vi "Convert file.vi"(8 "error in (no error)":errorcluster, 9 "file out":path, 10 "file in":path, 11 "DAQMH121119OrcaFlash in":refnum<class "DAQOrcaFlash.lvclass">) -> (0 "error out":errorcluster, 3 "DAQMH121119OrcaFlash out":refnum<class "DAQOrcaFlash.lvclass">)   [LabVIEW 2012, in "DAQOrcaFlash.lvclass"]
uses:
  DAQOrcaFlash.lvclass
  DAQOrcaFlash.lvclass/DAQOrcaFlash.ctl
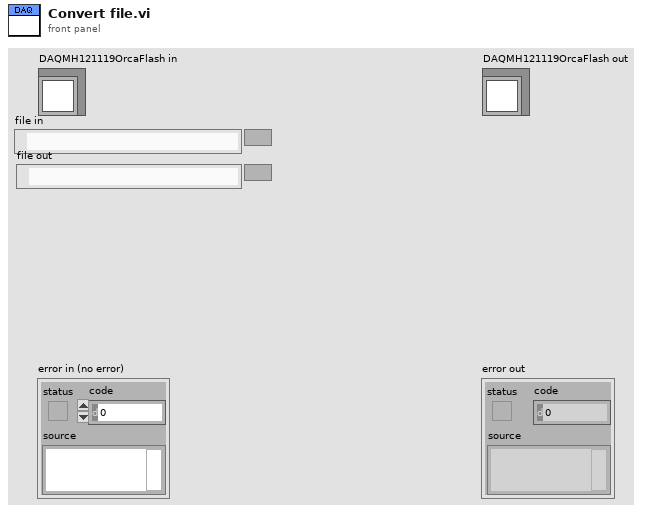
[diagram p1: front panel]
types:
  T1 = typedef "Image Type" = u32
  T2 = typedef "IMAQ Image.ctl" = refnum<image>
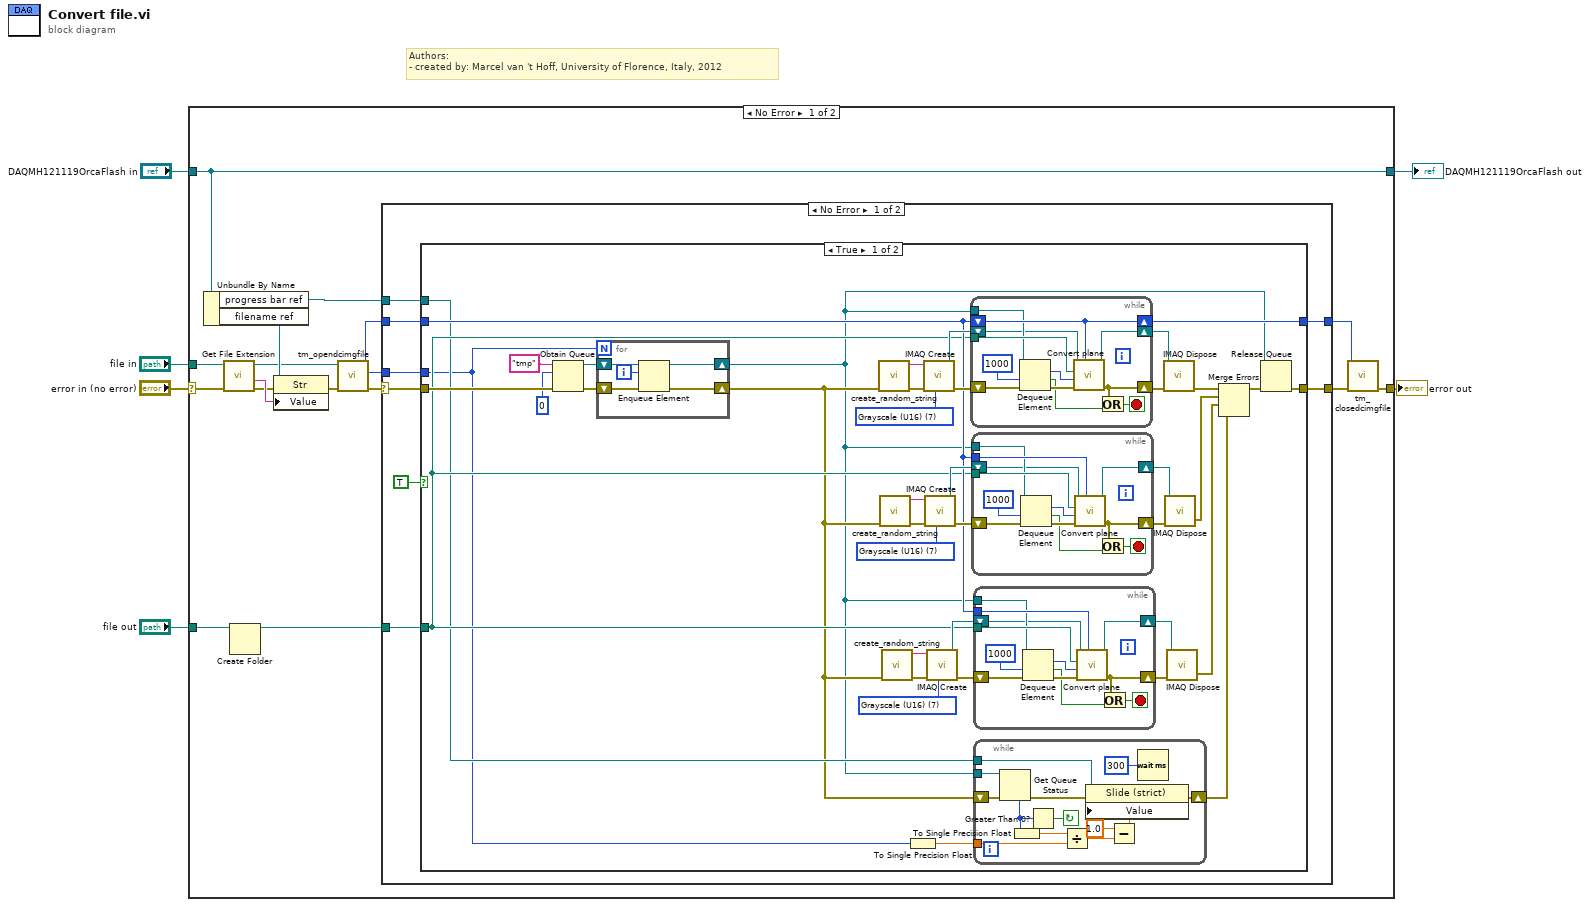
[diagram p0: block diagram]
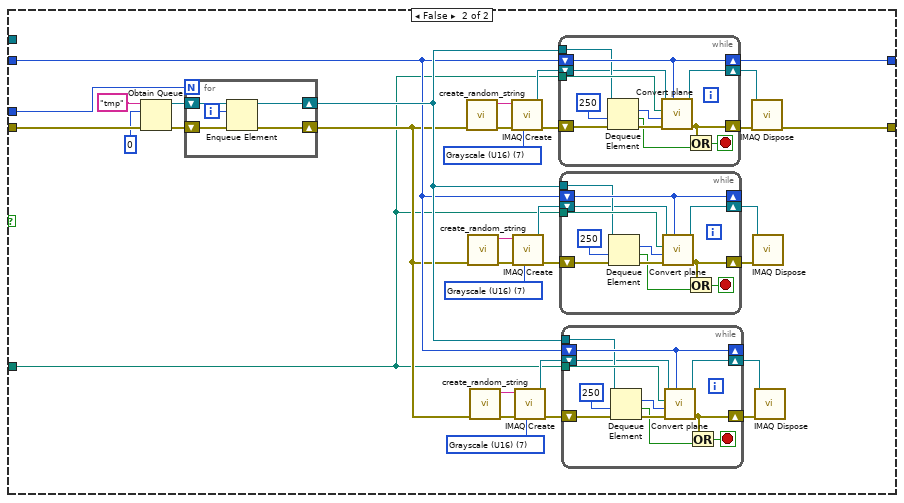
[diagram p2: hidden frame]
diagram:
  # "Authors: \n- created by: Marcel van 't Hoff, University of Florence, Italy, 2012"
  n1 = case shown="No Error" "error in (no error)" {
    selector: "error in (no error)" -> [w12 w203]
    tunnel: [w13 w203] -> w5
    tunnel: [w23 w202] -> w1
    tunnel: "DAQMH121119OrcaFlash in" -> [w23 w202]
    tunnel: "file in" -> [w11 _]
    tunnel: "file out" -> [w10 _]
    frame No Error {
      n2 = Unbundle By Name(w23) -> ("progress bar ref"=w19:refnum<vi>, "filename ref"=w22:refnum<vi>)
      n3 = call <vilib>:"Get File Extension.vi"("error in (no error)"=w12, "file"=w11) -> ("error out"=w20:errorcluster, "filename without extension"=w21:string, "dup file"=w7:path)  [unwired: 6 in, 1 out]
      n4 = Create Folder(path (use dialog)=w10) -> (created path=w9:path)  [unwired: 2 in, 2 out]
      n5 = property class="Str"(reference=w22, error in=w20, "Value"=w21) -> (error out=w8:errorcluster)  [unwired: 1 out]
      n6 = call <userlib>:"tm_opendcimgfile.vi"("error in (no error)"=w8, "Path"=w7) -> ("error out"=w16:errorcluster, "Total Frames"=w18:i32, "File Handle"=w17:u32)  [unwired: 7 in]
      n7 = case shown="No Error" w16 {
        selector: w16 -> [w31 w201]
        tunnel: w17 -> [w27 w200]
        tunnel: [w29 w201] -> w14
        tunnel: w18 -> [w28 _]
        tunnel: w9 -> [w26 _]
        tunnel: w19 -> [w24 _]
        tunnel: [w30 w200] -> w15
        frame No Error {
          n8 = case shown="True" TRUE {
            tunnel: w31 -> [w65 w152]
            tunnel: [w64 w151] -> w30
            tunnel: [w33 w150] -> w29
            tunnel: w28 -> [w40 w143]
            tunnel: w27 -> [w48 w132]
            tunnel: w26 -> [w47 w130]
            tunnel: w24 -> [w42 _]
            frame True {
              w50 = T1 7 items=["Grayscale (U8)", "Grayscale (I16)", "Grayscale (SGL)", "Complex (CSG)", "RGB (U32)", "HSL (U32)", "RGB (U64)", "Grayscale (U16)"] ("Image Type")
              w62 = T1 7 items=["Grayscale (U8)", "Grayscale (I16)", "Grayscale (SGL)", "Complex (CSG)", "RGB (U32)", "HSL (U32)", "RGB (U64)", "Grayscale (U16)"] ("Image Type")
              w67 = T1 7 items=["Grayscale (U8)", "Grayscale (I16)", "Grayscale (SGL)", "Complex (CSG)", "RGB (U32)", "HSL (U32)", "RGB (U64)", "Grayscale (U16)"] ("Image Type")
              n9 = Obtain Queue(name (unnamed)="tmp", element data type=0, error in (no error)=w65) -> (queue out=w43:refnum<queue>, error out=w46:errorcluster)  [unwired: 2 in, 1 out]
              n10 = for {
                N: w40 -> [_]
                shift-right: [w86] -> w41
                shift-left: w46 -> [w89]
                shift-right: [w85] -> w32
                shift-left: w43 -> [w88]
                i -> [w87]
                n11 = Enqueue Element(queue=w88, element=w87, error in (no error)=w89) -> (queue out=w85:refnum<queue>, error out=w86:errorcluster)  [unwired: 1 in, 1 out]
              }
              n12 = call "create_random_string.vi"("error in (no error)"=w41) -> ("error out"=w69:errorcluster, "random string"=w68:string)  [unwired: 9 in]
              n13 = call "create_random_string.vi"("error in (no error)"=w41) -> ("error out"=w60:errorcluster, "random string"=w61:string)  [unwired: 9 in]
              n14 = call "create_random_string.vi"("error in (no error)"=w41) -> ("error out"=w52:errorcluster, "random string"=w51:string)  [unwired: 9 in]
              n15 = To Single Precision Float(number=w40) -> (single precision float=w39:sgl)
              n16 = call "IMAQ Create"("Image Name"=w68, "Image Type"=w67, "error in (no error)"=w69) -> ("New Image"=w70:T2, "error out"=w66:errorcluster)  [unwired: 2 in]
              n17 = call "IMAQ Create"("Image Name"=w61, "Image Type"=w62, "error in (no error)"=w60) -> ("New Image"=w59:T2, "error out"=w63:errorcluster)  [unwired: 2 in]
              n18 = call "IMAQ Create"("Image Name"=w51, "Image Type"=w50, "error in (no error)"=w52) -> ("New Image"=w53:T2, "error out"=w49:errorcluster)  [unwired: 2 in]
              n19 = while {
                tunnel: w47 -> [w125]
                shift-right: [w116] -> w57
                shift-left: w66 -> [w121]
                shift-right: [w124] -> w71
                shift-left: w70 -> [w119]
                shift-right: [w123] -> w64
                shift-left: w48 -> [w123]
                tunnel: w32 -> [w122]
                stop <- w114 stop-if-true
                n20 = Dequeue Element(queue=w122, timeout in ms (-1)=1000, error in (no error)=w121) -> (element=w120:i32, timed out?=w115:bool, error out=w117:errorcluster)  [unwired: 1 out]
                n21 = call "Convert plane.vi"("File Handle"=w123, "error in (no error)"=w117, "Frame Index"=w120, "file in"=w125, "Image in"=w119) -> ("error out"=w116:errorcluster, "Image out"=w124:T2)  [unwired: 5 in]
                n22 = Or(x=w116, y=w115) -> (x .or. y?=w114:bool)
              }
              n23 = while {
                tunnel: w47 -> [w113]
                shift-right: [w102] -> w56
                shift-left: w63 -> [w109]
                shift-right: [w112] -> w58
                shift-left: w59 -> [w106]
                tunnel: w32 -> [w110]
                tunnel: w48 -> [w111]
                stop <- w103 stop-if-true
                n24 = Dequeue Element(queue=w110, timeout in ms (-1)=1000, error in (no error)=w109) -> (element=w107:i32, timed out?=w104:bool, error out=w108:errorcluster)  [unwired: 1 out]
                n25 = call "Convert plane.vi"("File Handle"=w111, "error in (no error)"=w108, "Frame Index"=w107, "file in"=w113, "Image in"=w106) -> ("error out"=w102:errorcluster, "Image out"=w112:T2)  [unwired: 5 in]
                n26 = Or(x=w102, y=w104) -> (x .or. y?=w103:bool)
              }
              n27 = while {
                tunnel: w47 -> [w101]
                shift-right: [w90] -> w55
                shift-left: w49 -> [w97]
                shift-right: [w100] -> w54
                shift-left: w53 -> [w94]
                tunnel: w32 -> [w98]
                tunnel: w48 -> [w99]
                stop <- w91 stop-if-true
                n28 = Dequeue Element(queue=w98, timeout in ms (-1)=1000, error in (no error)=w97) -> (element=w95:i32, timed out?=w92:bool, error out=w96:errorcluster)  [unwired: 1 out]
                n29 = call "Convert plane.vi"("File Handle"=w99, "error in (no error)"=w96, "Frame Index"=w95, "file in"=w101, "Image in"=w94) -> ("error out"=w90:errorcluster, "Image out"=w100:T2)  [unwired: 5 in]
                n30 = Or(x=w90, y=w92) -> (x .or. y?=w91:bool)
              }
              n31 = while {
                tunnel: w32 -> [w84]
                tunnel: w42 -> [w82]
                shift-right: [w79] -> w36
                shift-left: w41 -> [w80]
                tunnel: w39 -> [w77]
                stop <- w83 continue-if-true
                n32 = Get Queue Status(queue=w84, error in (no error)=w80) -> (error out=w81:errorcluster, # elements in queue=w78:i32)  [unwired: 1 in, 6 out]
                n33 = To Single Precision Float(number=w78) -> (single precision float=w76:sgl)
                n34 = Greater Than 0?(x=w78) -> (x > 0?=w83:bool)
                n35 = Divide(x=w76, y=w77) -> (x/y=w74:sgl)
                n36 = Subtract(x=sgl 1.0, y=w74) -> (x-y=w72:sgl)
                n37 = property class="Slide (strict)"(reference=w82, error in=w81, "Value"=w72) -> (error out=w79:errorcluster)  [unwired: 1 out]
                n38 = Wait (ms)(milliseconds to wait=u32 300) -> ()  [unwired: 1 out]
              }
              n39 = call "IMAQ Dispose"("Image"=w71, "error in (no error)"=w57) -> ("error out"=w35:errorcluster)  [unwired: 4 in]
              n40 = call "IMAQ Dispose"("Image"=w58, "error in (no error)"=w56) -> ("error out"=w38:errorcluster)  [unwired: 4 in]
              n41 = call "IMAQ Dispose"("Image"=w54, "error in (no error)"=w55) -> ("error out"=w37:errorcluster)  [unwired: 4 in]
              n42 = Merge Errors(w35, w38, w37, w36) -> (w34:errorcluster)
              n43 = Release Queue(queue=w32, error in (no error)=w34) -> (error out=w33:errorcluster)  [unwired: 1 in, 2 out]
            }
            frame False {
              w135 = T1 7 items=["Grayscale (U8)", "Grayscale (I16)", "Grayscale (SGL)", "Complex (CSG)", "RGB (U32)", "HSL (U32)", "RGB (U64)", "Grayscale (U16)"] ("Image Type")
              w148 = T1 7 items=["Grayscale (U8)", "Grayscale (I16)", "Grayscale (SGL)", "Complex (CSG)", "RGB (U32)", "HSL (U32)", "RGB (U64)", "Grayscale (U16)"] ("Image Type")
              w154 = T1 7 items=["Grayscale (U8)", "Grayscale (I16)", "Grayscale (SGL)", "Complex (CSG)", "RGB (U32)", "HSL (U32)", "RGB (U64)", "Grayscale (U16)"] ("Image Type")
              n44 = Obtain Queue(name (unnamed)="tmp", element data type=0, error in (no error)=w152) -> (queue out=w126:refnum<queue>, error out=w129:errorcluster)  [unwired: 2 in, 1 out]
              n45 = for {
                N: w143 -> [_]
                shift-right: [w160] -> w131
                shift-left: w129 -> [w163]
                shift-right: [w159] -> w133
                shift-left: w126 -> [w162]
                i -> [w161]
                n46 = Enqueue Element(queue=w162, element=w161, error in (no error)=w163) -> (queue out=w159:refnum<queue>, error out=w160:errorcluster)  [unwired: 1 in, 1 out]
              }
              n47 = call "create_random_string.vi"("error in (no error)"=w131) -> ("error out"=w156:errorcluster, "random string"=w155:string)  [unwired: 9 in]
              n48 = call "create_random_string.vi"("error in (no error)"=w131) -> ("error out"=w146:errorcluster, "random string"=w147:string)  [unwired: 9 in]
              n49 = call "create_random_string.vi"("error in (no error)"=w131) -> ("error out"=w137:errorcluster, "random string"=w136:string)  [unwired: 9 in]
              n50 = call "IMAQ Create"("Image Name"=w155, "Image Type"=w154, "error in (no error)"=w156) -> ("New Image"=w157:T2, "error out"=w153:errorcluster)  [unwired: 2 in]
              n51 = call "IMAQ Create"("Image Name"=w147, "Image Type"=w148, "error in (no error)"=w146) -> ("New Image"=w145:T2, "error out"=w149:errorcluster)  [unwired: 2 in]
              n52 = call "IMAQ Create"("Image Name"=w136, "Image Type"=w135, "error in (no error)"=w137) -> ("New Image"=w138:T2, "error out"=w134:errorcluster)  [unwired: 2 in]
              n53 = while {
                tunnel: w130 -> [w199]
                shift-right: [w190] -> w142
                shift-left: w153 -> [w195]
                shift-right: [w198] -> w158
                shift-left: w157 -> [w193]
                shift-right: [w197] -> w151
                shift-left: w132 -> [w197]
                tunnel: w133 -> [w196]
                stop <- w188 stop-if-true
                n54 = Dequeue Element(queue=w196, timeout in ms (-1)=250, error in (no error)=w195) -> (element=w194:i32, timed out?=w189:bool, error out=w191:errorcluster)  [unwired: 1 out]
                n55 = call "Convert plane.vi"("File Handle"=w197, "error in (no error)"=w191, "Frame Index"=w194, "file in"=w199, "Image in"=w193) -> ("error out"=w190:errorcluster, "Image out"=w198:T2)  [unwired: 5 in]
                n56 = Or(x=w190, y=w189) -> (x .or. y?=w188:bool)
              }
              n57 = while {
                tunnel: w130 -> [w187]
                shift-right: [w176] -> w141
                shift-left: w149 -> [w183]
                shift-right: [w186] -> w144
                shift-left: w145 -> [w180]
                shift-right: [w185] -> _
                shift-left: w132 -> [w185]
                tunnel: w133 -> [w184]
                stop <- w177 stop-if-true
                n58 = Dequeue Element(queue=w184, timeout in ms (-1)=250, error in (no error)=w183) -> (element=w181:i32, timed out?=w178:bool, error out=w182:errorcluster)  [unwired: 1 out]
                n59 = call "Convert plane.vi"("File Handle"=w185, "error in (no error)"=w182, "Frame Index"=w181, "file in"=w187, "Image in"=w180) -> ("error out"=w176:errorcluster, "Image out"=w186:T2)  [unwired: 5 in]
                n60 = Or(x=w176, y=w178) -> (x .or. y?=w177:bool)
              }
              n61 = while {
                tunnel: w130 -> [w175]
                shift-right: [w164] -> w140
                shift-left: w134 -> [w171]
                shift-right: [w174] -> w139
                shift-left: w138 -> [w168]
                shift-right: [w173] -> _
                shift-left: w132 -> [w173]
                tunnel: w133 -> [w172]
                stop <- w165 stop-if-true
                n62 = Dequeue Element(queue=w172, timeout in ms (-1)=250, error in (no error)=w171) -> (element=w169:i32, timed out?=w166:bool, error out=w170:errorcluster)  [unwired: 1 out]
                n63 = call "Convert plane.vi"("File Handle"=w173, "error in (no error)"=w170, "Frame Index"=w169, "file in"=w175, "Image in"=w168) -> ("error out"=w164:errorcluster, "Image out"=w174:T2)  [unwired: 5 in]
                n64 = Or(x=w164, y=w166) -> (x .or. y?=w165:bool)
              }
              n65 = call "IMAQ Dispose"("Image"=w158, "error in (no error)"=w142) -> ("error out"=w150:errorcluster)  [unwired: 4 in]
              n66 = call "IMAQ Dispose"("Image"=w144, "error in (no error)"=w141) -> ()  [unwired: 4 in, 1 out]
              n67 = call "IMAQ Dispose"("Image"=w139, "error in (no error)"=w140) -> ()  [unwired: 4 in, 1 out]
            }
          }
        }
        frame Error {
        }
      }
      n68 = call <userlib>:"tm_closedcimgfile.vi"("error in (no error)"=w14, "File Handle"=w15) -> ("error out"=w13:errorcluster)  [unwired: 9 in]
    }
    frame Error {
    }
  }
  "error out" <- w5
  "DAQMH121119OrcaFlash out" <- w1
